vi "KeyboardSimulation(String).vi"(0 "VI Reference In":refnum<vi>, 5 "String":string="Hello", 7 "Control Path":string, 11 "error In":errorcluster) -> (4 "VI Reference Out":refnum<vi>, 15 "error IO":errorcluster)   [LabVIEW 2016, in "Drona.lvlib"]
doc: "Simulates keyboard press for every letter in the input string."
uses:
  Drona.lvlib
  apis/Stimulus/KeyBoardSimulation/KeyboardSimulation.lvlib
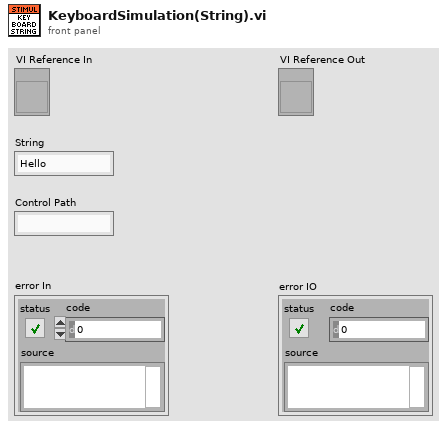
[diagram p1: front panel]
types:
  T1 = cluster{" Key":u8, "Action":enum16{"Press", "Up", "Down"}, "Delay (ms)":u32}
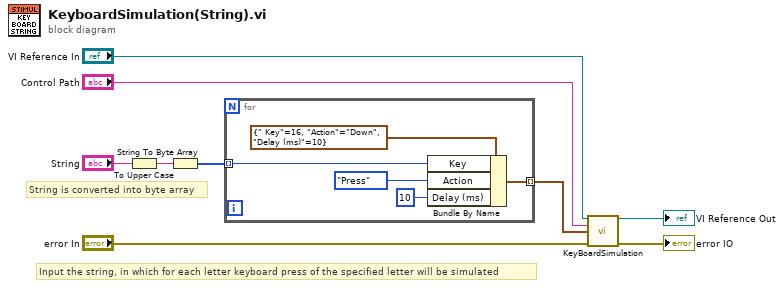
[diagram p0: block diagram]
diagram:
  # "Input the string, in which for each letter keyboard press of the specified letter will be simulated"
  # "String is converted into byte array"
  n1 = To Upper Case(1:"String") -> (0:w1:string)
  n2 = String To Byte Array(string=w1) -> (unsigned byte array=w9:u8[])
  n3 = for {
    tunnel: w9 -> [w11] mode=indexing
    tunnel: [w10] -> w8 mode=indexing
    n4 = Bundle By Name(cluster=T1 {" Key"=16, "Action"=enum."Down", "Delay (ms)"=10} ("Cluster"), "Key"=w11, "Action"=enum16{"Press", "Up", "Down"}."Press", "Delay (ms)"=u32 10) -> (w10:T1)
  }
  n5 = call "KeyBoardSimulation.vi"("VI Reference In"="VI Reference In", "Control Path"="Control Path", "Key Array"=w8, "error In"="error In") -> ("VI Reference Out"=→"VI Reference Out":refnum<vi>, "error IO"=→"error IO":errorcluster)  [unwired: 10 in]
